vi "dump.vi"(8 "error in (no error)":errorcluster, 10 "remove comments? (F)":bool, 11 "sections":T1[](array[typedef])) -> (0 "error out":errorcluster, 3 "toml":string)   [LabVIEW 2017, in "toml.lvlib"]
uses:
  toml.lvlib
  fg_section.ctl
  fg_row.ctl
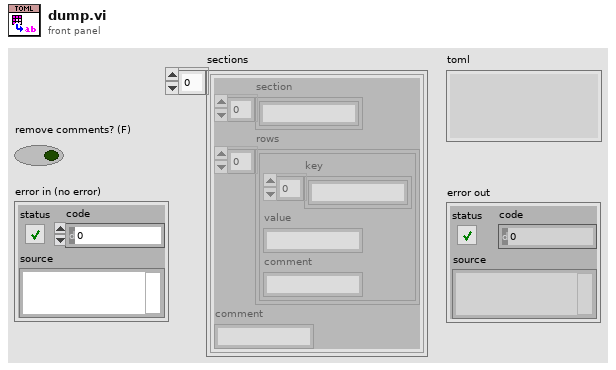
[diagram p1: front panel]
types:
  T1 = typedef "toml.lvlib/fg_section.ctl" = cluster{"section":string[], "rows":T2[], "comment":string}
  T2 = typedef "toml.lvlib/fg_row.ctl" = cluster{"key":string[], "value":string, "comment":string}
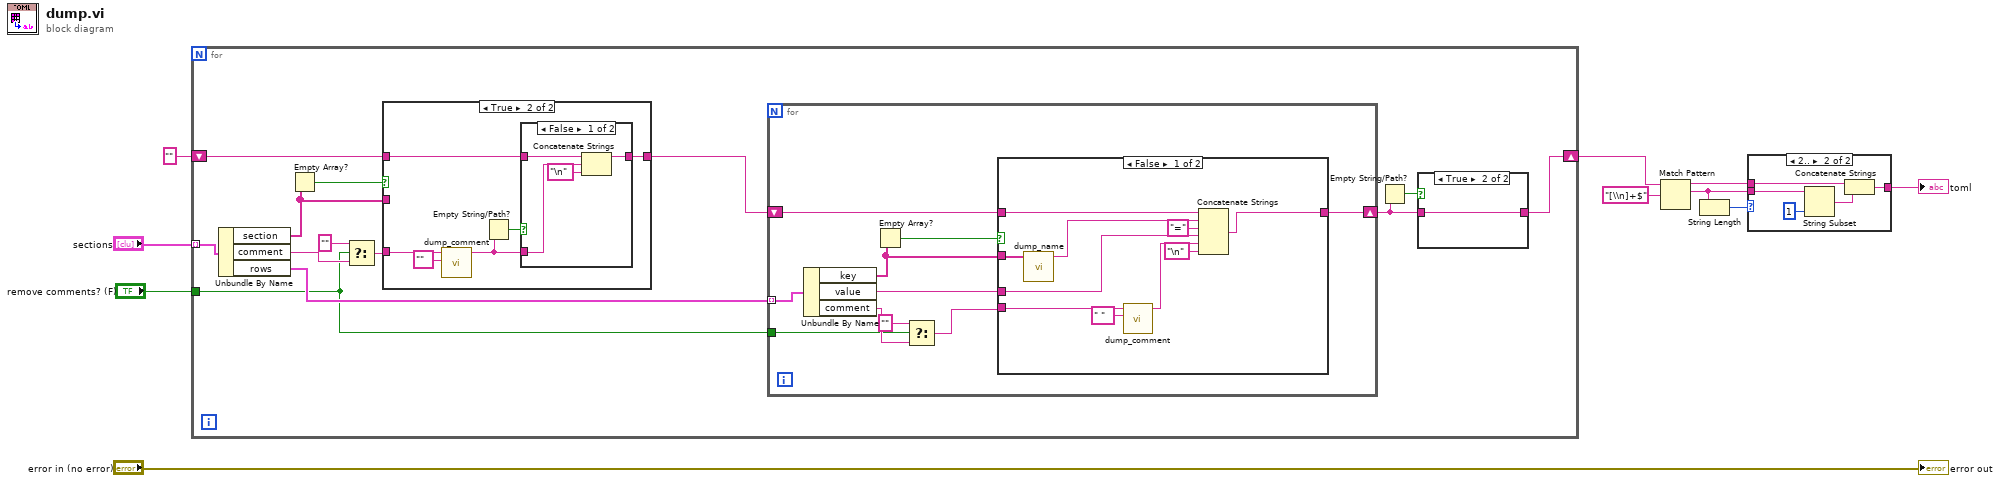
[diagram p0: block diagram]
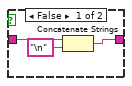
[diagram p3: hidden frame]
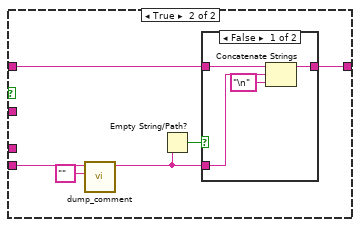
[diagram p4: hidden frame]
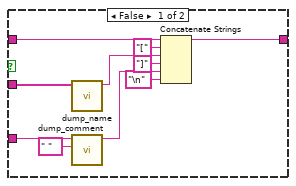
[diagram p6: hidden frame]
diagram:
  n1 = for {
    tunnel: "sections" -> [w23] mode=indexing
    shift-right: [w14] -> w5
    shift-left: "" -> [w21]
    tunnel: "remove comments? (F)" -> [w15]
    n2 = Unbundle By Name(w23) -> ("section"=w20:string[], "comment"=w17:string, "rows"=w19:T2[])
    n3 = Empty Array?(array=w20) -> (empty?=w22:bool)
    n4 = Select(t="", s=w15, f=w17) -> (s? t:f=w11:string)
    n5 = case shown="True" w22 {
      tunnel: [w66 w73] -> w18
      tunnel: w21 -> [w68 w74]
      tunnel: w20 -> [w67 _]
      tunnel: w11 -> [w61 w70]
      frame False {
        n6 = call "dump_name.vi"("section/key"=w67) -> ("toml"=w65:string)  [unwired: 10 in]
        n7 = call "dump_comment.vi"("left pad (\"\")"=" " ("left pad (\"\")"), "comment in"=w61) -> ("comment out"=w59:string)  [unwired: 9 in]
        n8 = Concatenate Strings(w68, "[" ("string"), w65, "]" ("string"), w59, "\n" ("string")) -> (w66:string)
      }
      frame True {
        n9 = call "dump_comment.vi"("left pad (\"\")"="" ("left pad (\"\")"), "comment in"=w70) -> ("comment out"=w69:string)  [unwired: 9 in]
        n10 = Empty String/Path?(string/path=w69) -> (empty?=w72:bool)
        n11 = case shown="False" w72 {
          tunnel: w74 -> [w78 w79]
          tunnel: [w77 w79] -> w73
          tunnel: w69 -> [w76 _]
          frame False {
            n12 = Concatenate Strings(w78, w76, "\n" ("string")) -> (w77:string)
          }
          frame True {
          }
        }
      }
    }
    n13 = for {
      tunnel: w19 -> [w33] mode=indexing
      shift-right: [w34] -> w13
      shift-left: w18 -> [w35]
      tunnel: w15 -> [w29]
      n14 = Unbundle By Name(w33) -> ("key"=w37:string[], "value"=w32:string, "comment"=w30:string)
      n15 = Empty Array?(array=w37) -> (empty?=w36:bool)
      n16 = Select(t="", s=w29, f=w30) -> (s? t:f=w28:string)
      n17 = case shown="False" w36 {
        tunnel: [w45 w52] -> w34
        tunnel: w35 -> [w47 w53]
        tunnel: w37 -> [w46 _]
        tunnel: w28 -> [w39 w49]
        tunnel: w32 -> [w41 _]
        frame False {
          n18 = call "dump_name.vi"("section/key"=w46) -> ("toml"=w44:string)  [unwired: 10 in]
          n19 = call "dump_comment.vi"("left pad (\"\")"=" " ("left pad (\"\")"), "comment in"=w39) -> ("comment out"=w38:string)  [unwired: 9 in]
          n20 = Concatenate Strings(w47, w44, "=" ("string"), w41, w38, "\n" ("string")) -> (w45:string)
        }
        frame True {
          n21 = call "dump_comment.vi"("left pad (\"\")"="" ("left pad (\"\")"), "comment in"=w49) -> ("comment out"=w48:string)  [unwired: 9 in]
          n22 = Empty String/Path?(string/path=w48) -> (empty?=w51:bool)
          n23 = case shown="False" w51 {
            tunnel: w53 -> [w57 w58]
            tunnel: [w56 w58] -> w52
            tunnel: w48 -> [w55 _]
            frame False {
              n24 = Concatenate Strings(w57, w55, "\n" ("string")) -> (w56:string)
            }
            frame True {
            }
          }
        }
      }
    }
    n25 = Empty String/Path?(string/path=w13) -> (empty?=w12:bool)
    n26 = case shown="True" w12 {
      tunnel: [w25 w27] -> w14
      tunnel: w13 -> [w24 w27]
      frame False {
        n27 = Concatenate Strings(w24, "\n" ("string")) -> (w25:string)
      }
      frame True {
      }
    }
  }
  n28 = Match Pattern(string=w5, regular expression="[\\n]+$" ("string")) -> (before substring=w4:string, match substring=w3:string)  [unwired: 1 in, 2 out]
  n29 = String Length(string=w3) -> (length=w1:i32)
  n30 = case shown="2.." w1 {
    tunnel: w4 -> [w80 w85]
    tunnel: w3 -> [_ w84]
    tunnel: [w80 w82] -> w2
    frame ..1 {
    }
    frame 2.. {
      n31 = String Subset(string=w84, length (rest)=1 ("length (rest)")) -> (substring=w81:string)  [unwired: 1 in]
      n32 = Concatenate Strings(w85, w81) -> (w82:string)
    }
  }
  "toml" <- w2
  "error out" <- "error in (no error)"
